vi "topVI.vi"() -> ()   [LabVIEW 2014]
panel:
  out "resistance total num":u32
  out "color total num":u32
  out "resistance correct num":u32
  out "color correct num":u32
  out "Answear Time (sec) 2":dbl
  out "Correct or not? 2":bool
  out "Answear Time (sec)":dbl
  out "Correct or not?":bool
  in  "stop":bool
  in  "Menu cluster":cluster{bool, bool, bool}
  # "電阻色碼練習遊戲"
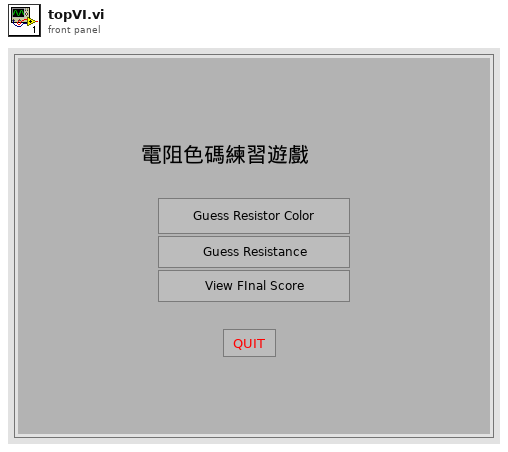
[diagram p1: front panel]
types:
  T1 = enum16{"idle", "guess_color", "guess_resistance", "view_score"}
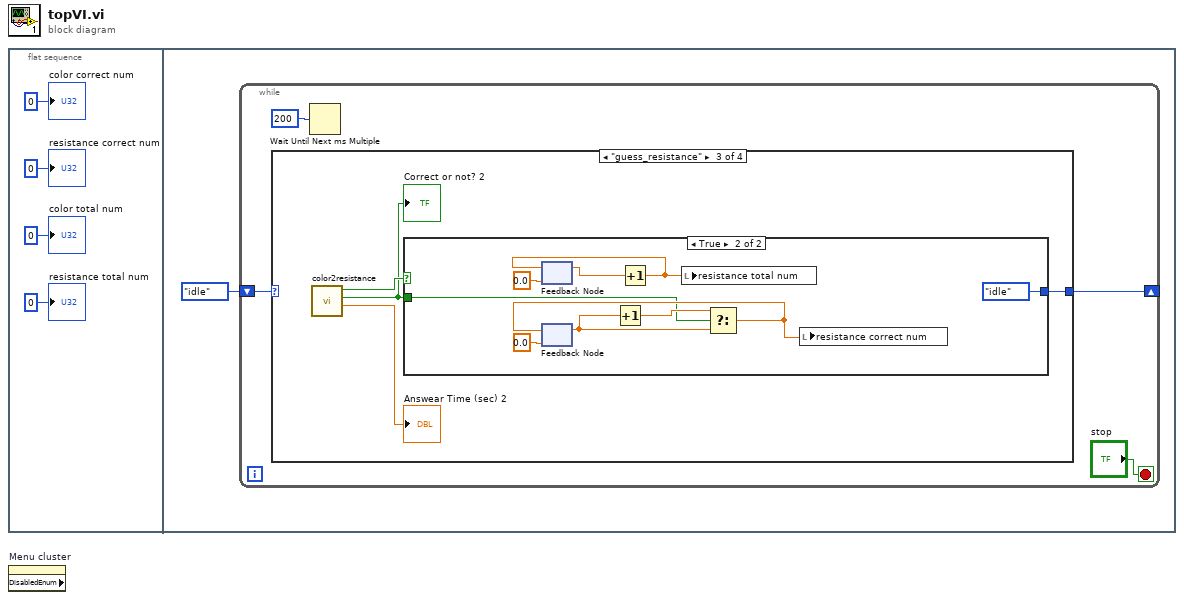
[diagram p0: block diagram]
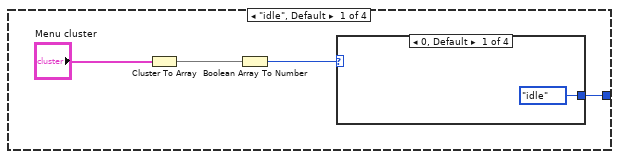
[diagram p2: hidden frame]
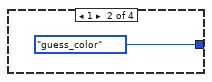
[diagram p3: hidden frame]
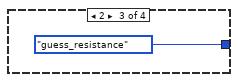
[diagram p4: hidden frame]
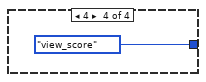
[diagram p5: hidden frame]
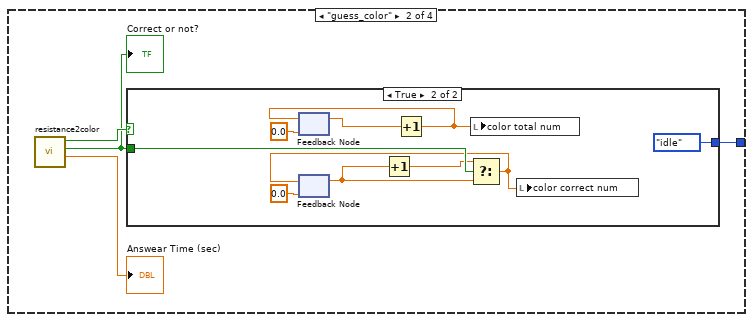
[diagram p6: hidden frame]
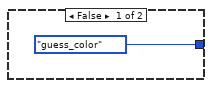
[diagram p7: hidden frame]
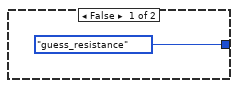
[diagram p8: hidden frame]
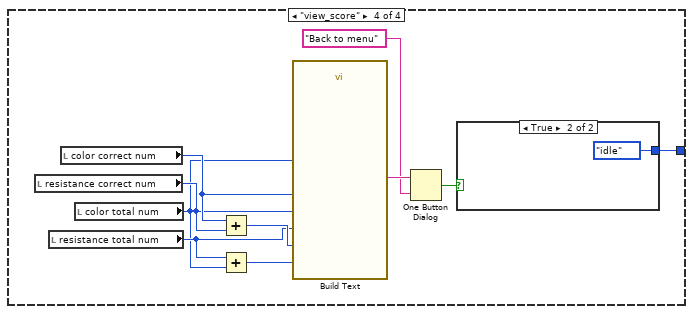
[diagram p9: hidden frame]
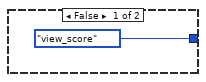
[diagram p10: hidden frame]
diagram:
  n1 = flat-sequence {
    frame #0 {
      "color correct num" <- u32 0 ("color correct num")
      "resistance correct num" <- u32 0 ("resistance correct num")
      "color total num" <- u32 0 ("color correct num")
      "resistance total num" <- u32 0 ("resistance correct num")
    }
    frame #1 {
      n2 = while {
        shift-right: [w7] -> _
        shift-left: T1."idle" -> [w8]
        stop <- "stop" stop-if-true
        n3 = case shown="\"guess_resistance\"" w8 {
          tunnel: [w11 w21 w35 w55] -> w7
          frame "idle", Default {
            n4 = Cluster To Array(cluster="Menu cluster") -> (array=w12:bool[])
            n5 = Boolean Array To Number(Boolean array=w12) -> (number=w10:u32)
            n6 = case shown="0, Default" w10 {
              tunnel: [T1."idle" T1."guess_color" T1."guess_resistance" T1."view_score"] -> w11
              frame 0, Default {
              }
              frame 1 {
              }
              frame 2 {
              }
              frame 4 {
              }
            }
          }
          frame "guess_color" {
            n7 = call "resistance2color.vi"() -> ("Finish"=w19:bool, "Correct or not?"=w18:bool, "Answear Time (sec)"=→"Answear Time (sec)":dbl)  [unwired: 6 in]
            "Correct or not?" <- w18
            n8 = case shown="True" w19 {
              tunnel: [T1."guess_color" T1."idle"] -> w21
              tunnel: w18 -> [_ w30]
              frame False {
              }
              frame True {
                n9 = feedback #1(0.0) -> (w26:dbl)
                n10 = feedback #2(0.0) -> (w28:dbl)
                n11 = Increment(x=w28) -> (x+1=w27:dbl)
                n12 = Increment(x=w26) -> (x+1=w23:dbl)
                n13 = feedback-in #1(w23) -> ()
                n14 = local write "color total num"(w23) -> ()
                n15 = Select(t=w27, s=w30, f=w28) -> (s? t:f=w29:dbl)
                n16 = feedback-in #2(w29) -> ()
                n17 = local write "color correct num"(w29) -> ()
              }
            }
          }
          frame "guess_resistance" {
            n18 = call "color2resistance.vi"() -> ("finish"=w33:bool, "Correct or not"=w32:bool, "Answear Time (sec)"=→"Answear Time (sec) 2":dbl)  [unwired: 6 in]
            "Correct or not? 2" <- w32
            n19 = case shown="True" w33 {
              tunnel: [T1."guess_resistance" T1."idle"] -> w35
              tunnel: w32 -> [_ w37]
              frame False {
              }
              frame True {
                n20 = feedback #3(0.0) -> (w41:dbl)
                n21 = feedback #4(0.0) -> (w43:dbl)
                n22 = Increment(x=w43) -> (x+1=w42:dbl)
                n23 = Increment(x=w41) -> (x+1=w38:dbl)
                n24 = feedback-in #3(w38) -> ()
                n25 = local write "resistance total num"(w38) -> ()
                n26 = Select(t=w42, s=w37, f=w43) -> (s? t:f=w44:dbl)
                n27 = feedback-in #4(w44) -> ()
                n28 = local write "resistance correct num"(w44) -> ()
              }
            }
          }
          frame "view_score" {
            n29 = local read "resistance correct num"() -> (w49:u32)
            n30 = local read "resistance total num"() -> (w47:u32)
            n31 = local read "color correct num"() -> (w50:u32)
            n32 = local read "color total num"() -> (w46:u32)
            n33 = Add(x=w50, y=w49) -> (x+y=w51:u32)
            n34 = Add(x=w47, y=w46) -> (x+y=w48:u32)
            n35 = call "Build Text"("resistance_total"=w47, "total"=w48, "color_correct"=w50, "color_total"=w46, "resistance_correct"=w49, "correct"=w51) -> ("Result"=w54:string)  [unwired: 8 in, 1 out]
            n36 = One Button Dialog(message=w54, button name ("OK")="Back to menu") -> (true=w52:bool)
            n37 = case shown="True" w52 {
              tunnel: [T1."view_score" T1."idle"] -> w55
              frame False {
              }
              frame True {
              }
            }
          }
        }
        n38 = Wait Until Next ms Multiple(millisecond multiple=u32 200) -> ()  [unwired: 1 out]
      }
    }
  }
  n39 = property on="Menu cluster" class="Clust" props=["DisabledEnum"]() -> ()  [unwired: 2 in, 3 out]
